vi "Launch.vi"(5 "window position":cluster{"Left":i16, "Top":i16}, 7 "options":T1, 8 "error in (no error)":errorcluster, 11 "Thread in":refnum<class "Thread.lvclass">) -> (0 "error out":errorcluster, 3 "Thread out":refnum<class "Thread.lvclass">)   [LabVIEW 2021, in "DSF Core.lvlib" / "Thread.lvclass"]
uses:
  Thread.lvclass
  Thread Options.ctl
  Thread.lvclass/Thread.ctl
  Top.vi
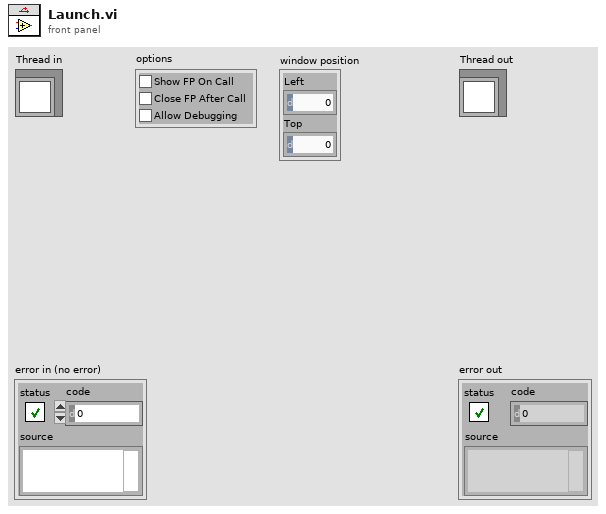
[diagram p1: front panel]
types:
  T1 = typedef "DSF Core.lvlib/Thread.lvclass/Thread Options.ctl" = cluster{"Show FP On Call":bool, "Close FP After Call":bool, "Allow Debugging":bool}
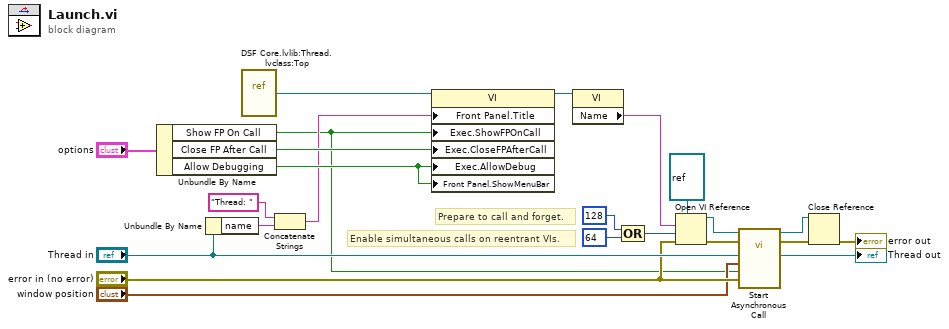
[diagram p0: block diagram]
diagram:
  # "Prepare to call and forget."
  # "Enable simultaneous calls on reentrant VIs."
  n1 = Unbundle By Name("options") -> ("Show FP On Call"=w1:bool, "Close FP After Call"=w16:bool, "Allow Debugging"=w11:bool)
  n2 = Unbundle By Name("Thread in") -> ("name"=w14:string)
  n3 = vi-ref "DSF Core.lvlib:Thread.lvclass:Top.vi"() -> (w13:refnum<vi>)
  n4 = Concatenate Strings("Thread: " ("string"), w14) -> (w10:string)
  n5 = property class="VI"(reference=w13, "Front Panel.Title"=w10, "Exec.ShowFPOnCall"=w1, "Exec.CloseFPAfterCall"=w16, "Exec.AllowDebug"=w11, "Front Panel.ShowMenuBar"=w11) -> (reference out=w18:refnum<vi>)  [unwired: 1 in, 1 out]
  n6 = property class="VI"(reference=w18) -> ("Name"=w12:string)  [unwired: 1 in, 2 out]
  n7 = Compound Arithmetic op=OR(128 ("options"), 64 ("options")) -> (w19:i32)
  n8 = Open VI Reference(type specifier VI Refnum (for type only)=refnum<vi> refnum, vi path=w12, options=w19, error in (no error)="error in (no error)") -> (vi reference=w2:refnum<vi>, error out=w3:errorcluster)  [unwired: 2 in]
  n9 = call-by-ref "Start Asynchronous Call"(reference=w2, error in=w3, 8:"error in (no error)"="error in (no error)", "reposition window"=w1, "window position"="window position", "Thread in"="Thread in") -> (reference out=w6:refnum<vi>, error out=w8:errorcluster)  [unwired: 6 in, 2 out]
  n10 = Close Reference(reference=w6, error in (no error)=w8) -> (error out=→"error out":errorcluster)
  "Thread out" <- "Thread in"
